vi "unc_combine.vi"(1 "k":dbl=1.0, 2 "ua":cdb, 3 "ub":cdb) -> (0 "uc":cdb)   [LabVIEW 2020, in "varilib.lvlib"]
doc: "Combine two standard uncerainties, eventually expand by coefficient 'k'.\nIt works with complex numbers as well."
uses:
  varilib.lvlib
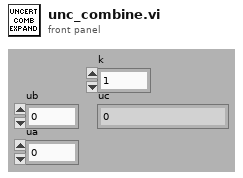
[diagram p1: front panel]
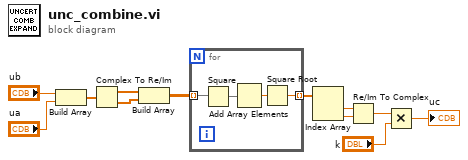
[diagram p0: block diagram]
diagram:
  n1 = Build Array("ub", "ua") -> (w10:cdb[])
  n2 = Complex To Re/Im(x + iy=w10) -> (x=w9:dbl[], y=w8:dbl[])
  n3 = Build Array(w9, w8) -> (w7:dbl[][])
  n4 = for {
    tunnel: w7 -> [w16] mode=indexing
    tunnel: [w13] -> w6 mode=indexing
    n5 = Square(x=w16) -> (x^2=w15:dbl[])
    n6 = Add Array Elements(numeric array=w15) -> (sum=w14:dbl)
    n7 = Square Root(x=w14) -> (sqrt(x)=w13:dbl)
  }
  n8 = Index Array(array=w6) -> (element #1=w5:dbl, element #2=w4:dbl)  [unwired: 2 in]
  n9 = Re/Im To Complex(1:w4, 2:w5) -> (0:w3:cdb)
  n10 = Multiply(x=w3, y="k") -> (x*y=→"uc":cdb)
